vi "DQtoABC_noSine_PowInv.vi"(0 "direct":sgl format="%#_30g", 1 "cosx":sgl, 2 "sinx":sgl, 5 "quadrature":sgl format="%#_30g", 12 "Resources":T1) -> (4 "A":sgl format="%#_32g", 6 "B":sgl, 8 "C":sgl, 10 "alpha":sgl format="%#_30g", 15 "beta":sgl format="%#_30g")   [LabVIEW 2017]
uses:
  Multiplier/Multiplier.lvclass
  Adder/Adder.lvclass
  Subtractor/Subtractor.lvclass
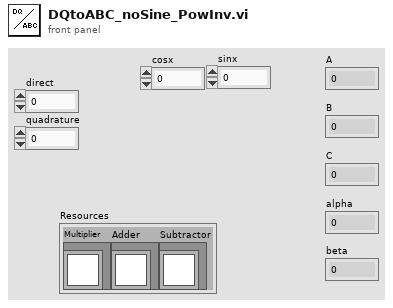
[diagram p1: front panel]
types:
  T1 = cluster{"Multiplier":refnum<class "Multiplier.lvclass">, "Adder":refnum<class "Adder.lvclass">, "Subtractor":refnum<class "Subtractor.lvclass">}
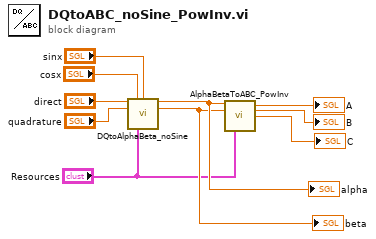
[diagram p0: block diagram]
diagram:
  n1 = call "DQtoAlphaBeta_noSine.vi"("direct"="direct", "cosx"="cosx", "sinx"="sinx", "quadrature"="quadrature", "Resources"="Resources") -> ("alpha"=w7:sgl, "beta"=w6:sgl)  [unwired: 9 in]
  "alpha" <- w7
  "beta" <- w6
  n2 = call "AlphaBetaToABC_PowInv.vi"("alpha"=w7, "beta"=w6, "Resources"="Resources") -> ("A"=→"A":sgl, "B"=→"B":sgl, "C"=→"C":sgl)  [unwired: 10 in]
